vi "Enqueue Element.vi"(6 "High Priority?(F)":bool, 8 "error in (no error)":errorcluster, 9 "timeout in ms (-1)":i32, 10 "Cross JKI State Machine State":T1, 11 "Priority Queue":refnum<class "Priority Queue.lvclass">) -> (0 "error out":errorcluster, 3 "Priority Queue(dup)":refnum<class "Priority Queue.lvclass">)   [LabVIEW 2020, in "Communicable State Machine.lvlib" / "Priority Queue.lvclass"]
uses:
  Priority Queue.lvclass
  _Cross CSM State Data.ctl
  _CSM_MSG_TYPE.ctl
  _Cross CSM State Response.ctl
  _CSM_Response Source Message.ctl
  Priority Queue.lvclass/Priority Queue.ctl
  def-Data(LowPRI-Q).ctl
  Communicable State Machine.lvlib
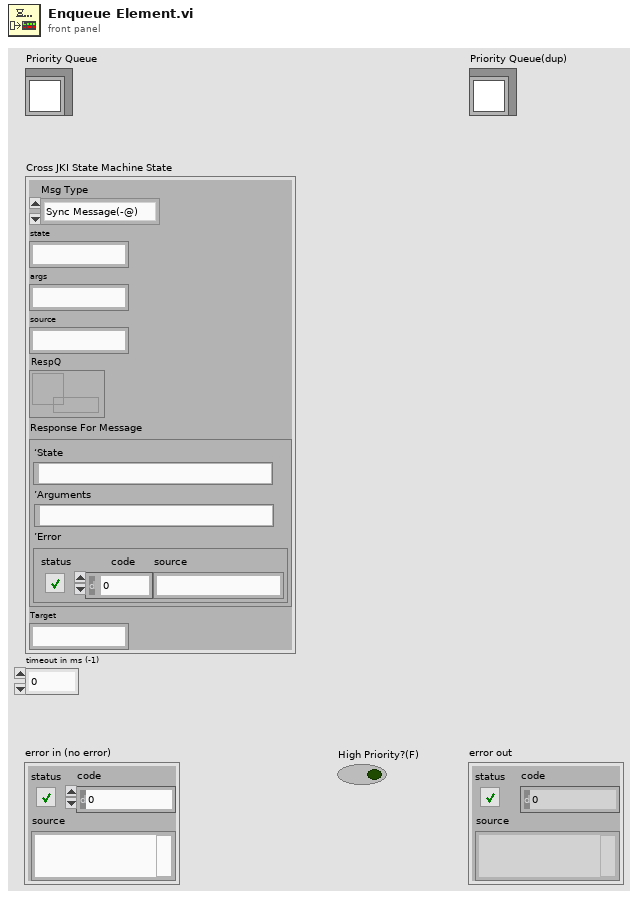
[diagram p1: front panel]
types:
  T1 = typedef "Communicable State Machine.lvlib/_Cross CSM State Data.ctl" = cluster{"Msg Type":T2, "state":string, "args":string, "source":string, "RespQ":refnum<queue>, "Response For Message":T3, "Target":string}
  T2 = typedef "Communicable State Machine.lvlib/_CSM_MSG_TYPE.ctl" = enum16{"Sync Message(-@)", "Async Message(->)", "Async without Response(->|)", "Async Response", "Broadcast(-><all>)", "Broadcast(-><status>)", "Broadcast(-><interrupt>)", "Append to JKISM States", "Append to JKISM States(High Priority)"}
  T3 = typedef "Communicable State Machine.lvlib/_CSM_Response Source Message.ctl" = cluster{"‘State":string, "’Arguments":string, "’Error":errorcluster}
  T4 = typedef "Communicable State Machine.lvlib/Priority Queue.lvclass/def-Data(LowPRI-Q).ctl" = cluster{"Data":T1, "Notify?":bool}
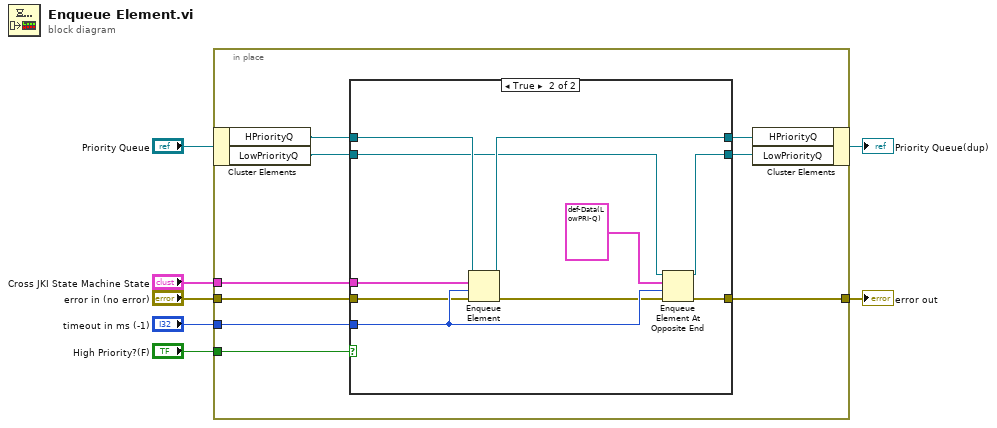
[diagram p0: block diagram]
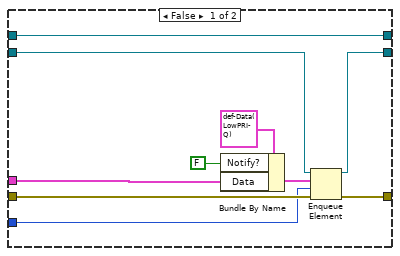
[diagram p2: hidden frame]
diagram:
  n1 = in-place {
    in-place-border: [w16] -> w7
    in-place-border: "error in (no error)" -> [w15]
    in-place-border: "High Priority?(F)" -> [w14]
    in-place-border: "Cross JKI State Machine State" -> [w13]
    in-place-border: "timeout in ms (-1)" -> [w12]
    n2 = in-place-cluster #1("Priority Queue") -> ("HPriorityQ"=w10:refnum<queue>, "LowPriorityQ"=w9:refnum<queue>)
    n3 = case shown="True" w14 {
      tunnel: w13 -> [w22 w36]
      tunnel: w15 -> [w26 w33]
      tunnel: [w25 w35] -> w16
      tunnel: w12 -> [w24 w34]
      tunnel: [w20 w29] -> w11
      tunnel: w10 -> [w20 w30]
      tunnel: w9 -> [w18 w28]
      tunnel: [w17 w27] -> w8
      frame False {
        n4 = Bundle By Name(cluster=T4 {"Data"={"Msg Type"=enum."Sync Message(-@)", "state"="", "args"="", "source"="", "RespQ"=refnum, "Response For Message"={"‘State"="", "’Arguments"="", "’Error"={"status"=FALSE, "code"=0, "source"=""}}, "Target"=""}, "Notify?"=FALSE}, "Notify?"=FALSE, "Data"=w22) -> (w21:T4)
        n5 = Enqueue Element(queue=w18, element=w21, timeout in ms (-1)=w24, error in (no error)=w26) -> (queue out=w17:refnum<queue>, error out=w25:errorcluster)  [unwired: 1 out]
      }
      frame True {
        n6 = Enqueue Element(queue=w30, element=w36, timeout in ms (-1)=w34, error in (no error)=w33) -> (queue out=w29:refnum<queue>, error out=w32:errorcluster)  [unwired: 1 out]
        n7 = Enqueue Element At Opposite End(queue=w28, element=T4 {"Data"={"Msg Type"=enum."Sync Message(-@)", "state"="", "args"="", "source"="", "RespQ"=refnum, "Response For Message"={"‘State"="", "’Arguments"="", "’Error"={"status"=FALSE, "code"=0, "source"=""}}, "Target"=""}, "Notify?"=TRUE} ("cluster"), timeout in ms (-1)=w34, error in (no error)=w32) -> (queue out=w27:refnum<queue>, error out=w35:errorcluster)  [unwired: 1 out]
      }
    }
    n8 = in-place-cluster #1("HPriorityQ"=w11, "LowPriorityQ"=w8) -> (→"Priority Queue(dup)":refnum<class "Priority Queue.lvclass">)
  }
  "error out" <- w7
